vi "Timer.vi"(8 "error in (no error)":errorcluster, 9 "Time Target(s)":dbl, 10 "Reset":bool, 11 "Pause":bool) -> (0 "error out":errorcluster, 1 "Elpased Time":dbl, 2 "Elapsed?":bool)   [LabVIEW 2013]
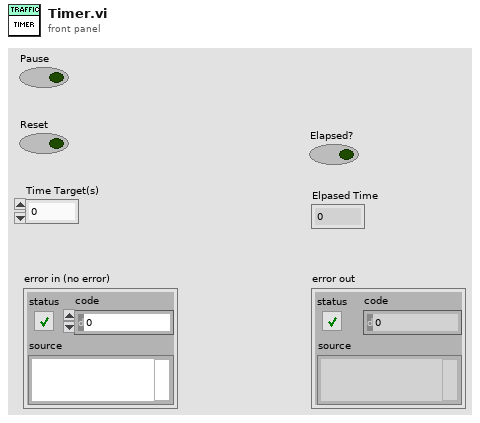
[diagram p1: front panel]
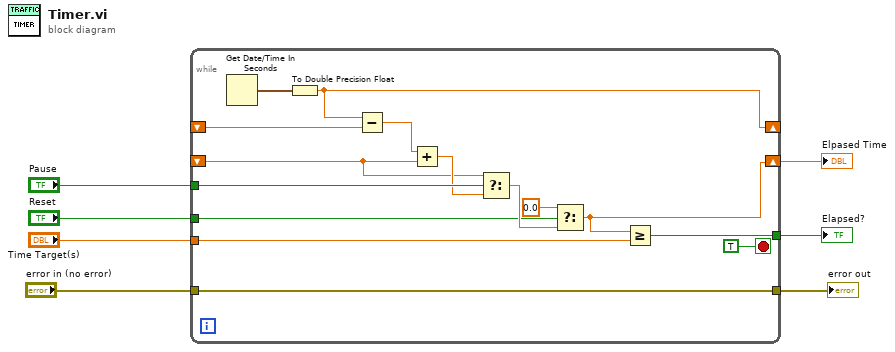
[diagram p0: block diagram]
diagram:
  n1 = while {
    shift-right: [w21] -> _
    shift-left: _ -> [w20]
    shift-right: [w12] -> w7
    shift-left: _ -> [w10]
    tunnel: "Pause" -> [w18]
    tunnel: "Reset" -> [w15]
    tunnel: "Time Target(s)" -> [w13]
    tunnel: [w11] -> w6
    tunnel: [w8] -> w2
    tunnel: "error in (no error)" -> [w8]
    stop <- TRUE stop-if-true
    n2 = Get Date/Time In Seconds() -> (seconds since 1Jan1904=w22:timestamp)
    n3 = To Double Precision Float(number=w22) -> (double precision float=w21:dbl)
    n4 = Subtract(x=w21, y=w20) -> (x-y=w19:dbl)
    n5 = Add(x=w19, y=w10) -> (x+y=w17:dbl)
    n6 = Select(t=w10, s=w18, f=w17) -> (s? t:f=w16:dbl)
    n7 = Select(t=0.0, s=w15, f=w16) -> (s? t:f=w12:dbl)
    n8 = Greater Or Equal?(x=w12, y=w13) -> (x >= y?=w11:bool)
  }
  "Elpased Time" <- w7
  "Elapsed?" <- w6
  "error out" <- w2
